vi "Get ClassItems from ProjectItem.vi"(8 "error in (no error)":errorcluster, 11 "ProjectItem in":refnum<vi>) -> (0 "error out":errorcluster, 1 "Class Item Names":string[](array[string]), 2 "Class Items":refnum<vi>[](array[refnum]), 3 "ProjectItem out":refnum<vi>)   [LabVIEW 2020, in "gRPC Scripting Tools.lvlib"]
uses:
  gRPC Scripting Tools.lvlib
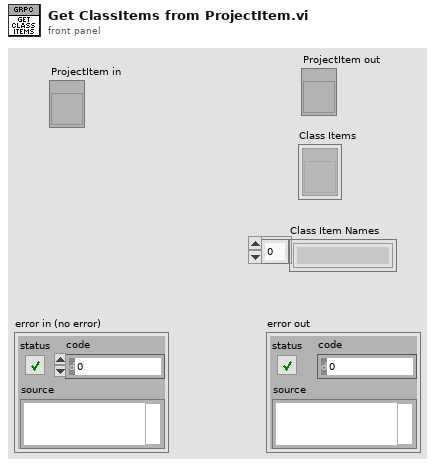
[diagram p1: front panel]
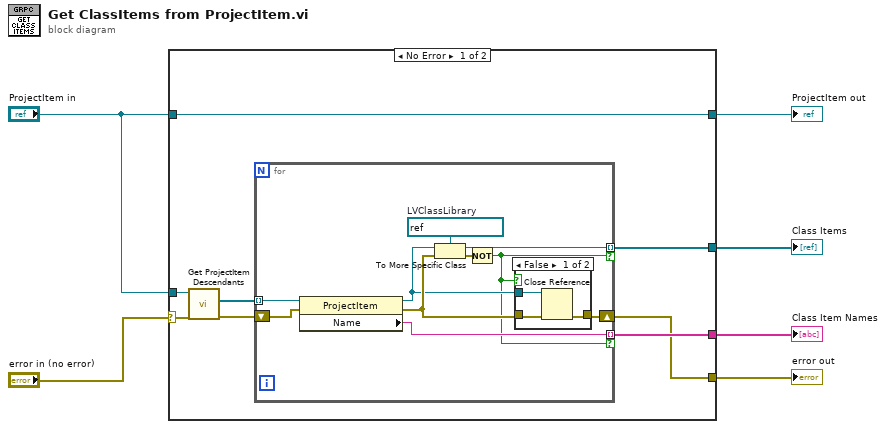
[diagram p0: block diagram]
diagram:
  n1 = case shown="No Error" "error in (no error)" {
    selector: "error in (no error)" -> [w7 w29]
    tunnel: "ProjectItem in" -> [w14 _]
    tunnel: [w12 _] -> w6
    tunnel: [w10 _] -> w5
    tunnel: [w9 w29] -> w4
    tunnel: "ProjectItem in" -> [w8 w30]
    tunnel: [w8 w30] -> w2
    frame No Error {
      n2 = call "Get ProjectItem Descendants.vi"("error in (no error)"=w7, "ProjectItem in"=w14) -> ("error out"=w13:errorcluster, "All Descendents"=w11:refnum<vi>[])  [unwired: 7 in, 1 out]
      n3 = for {
        tunnel: w11 -> [w24] mode=indexing
        tunnel: [w23] -> w12 mode=indexing if=w15
        tunnel: [w20] -> w10 mode=indexing if=w15
        shift-right: [w17] -> w9
        shift-left: w13 -> [w19]
        w22 = refnum<vi> refnum  # LVClassLibrary
        n4 = property class="ProjectItem"(reference=w24, error in=w19) -> (reference out=w16:refnum<vi>, error out=w18:errorcluster, "Name"=w23:string)
        n5 = To More Specific Class(target class=w22, reference=w16, error in=w18) -> (specific class reference=w20:refnum<vi>, error out=w21:errorcluster)
        n6 = Not(x=w21) -> (.not. x?=w15:bool)
        n7 = case shown="False" w15 {
          tunnel: w18 -> [w27 w28]
          tunnel: [w26 w28] -> w17
          tunnel: w16 -> [w25 _]
          frame False {
            n8 = Close Reference(reference=w25, error in (no error)=w27) -> (error out=w26:errorcluster)
          }
          frame True {
          }
        }
      }
    }
    frame Error {
    }
  }
  "Class Item Names" <- w6
  "Class Items" <- w5
  "ProjectItem out" <- w2
  "error out" <- w4
